vi "DBTableToTree.vi"(7 "NetworkName":string, 8 "error in (no error)":errorcluster, 9 "DBNode":T1(array[cluster]), 10 "DBSignals":T3(array[cluster]) {"SignalList"."Message_Type" items=["CAN", "CANFD", "J1939"]; "SignalList"."Mux_Type" items=["Normal", "multiplexor", "multiplexed"]; "SignalList"."Is_Motorola" items=["Intel", "Motorola"]; "SignalList"."Value_Type" items=["unsigned int", "signed int", "float", "double"]; "SignalList"."ID" format="%.0x"}, 11 "reference":refnum<vi>) -> (0 "error out":errorcluster)   [LabVIEW 2014]
uses:
  Typedef/DBSignal.ctl
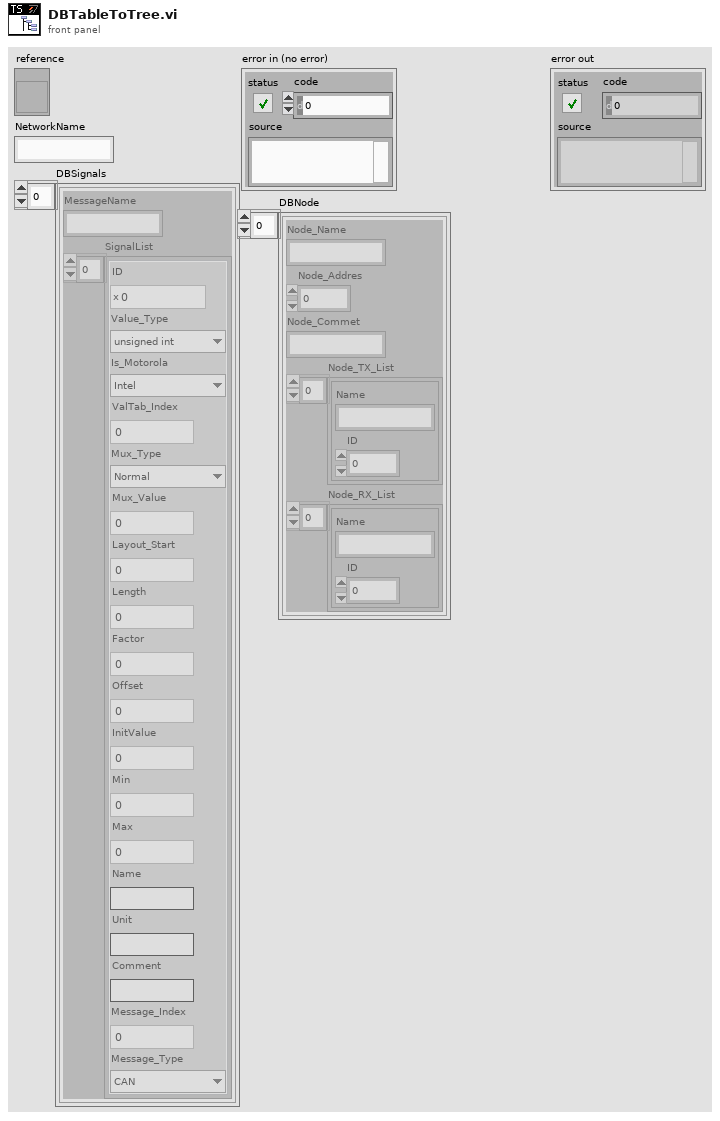
[diagram p1: front panel]
types:
  T1 = cluster{"Node_Name":string, "Node_Addres":i32, "Node_Commet":string, "Node_TX_List":cluster{"Name":string, "ID":i32}[], "Node_RX_List":cluster{"Name":string, "ID":i32}[]}[]
  T2 = typedef "DBSignal.ctl" = cluster{"ID":i32, "Value_Type":i32, "Is_Motorola":i32, "ValTab_Index":i32, "Mux_Type":i32, "Mux_Value":dbl, "Layout_Start":i32, "Length":i32, "Factor":dbl, "Offset":dbl, "InitValue":dbl, "Min":dbl, "Max":dbl, "Name":string, "Unit":string, "Comment":string, "Message_Index":i32, "Message_Type":i32}
  T3 = cluster{"MessageName":string, "SignalList":T2[]}[]
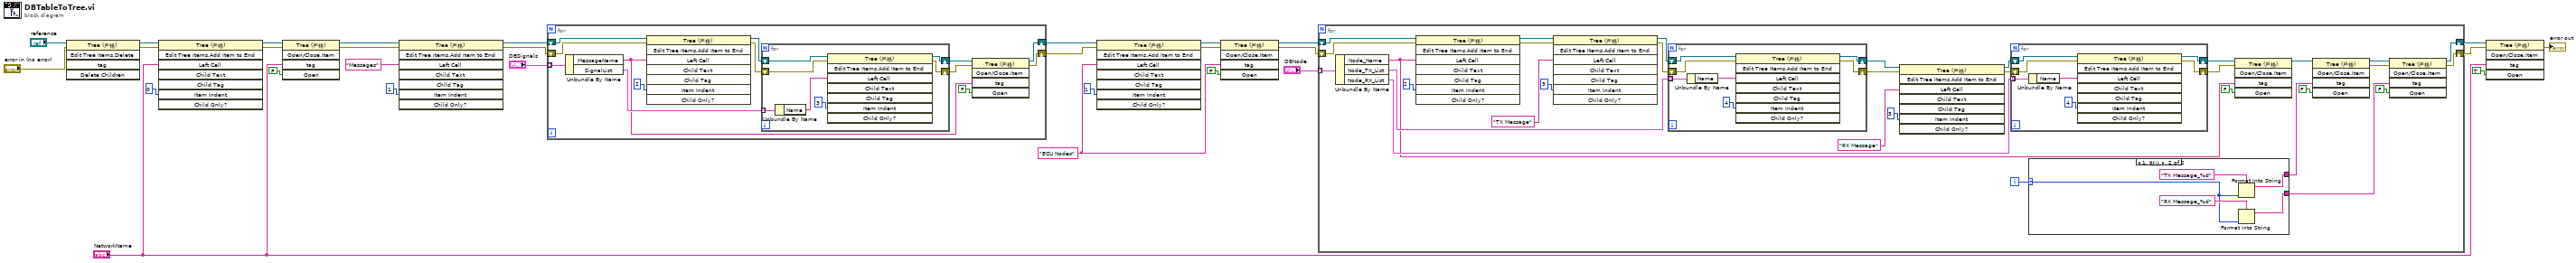
[diagram p0: block diagram]
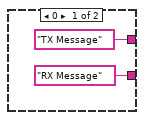
[diagram p2: hidden frame]
diagram:
  w4 = "ECU Nodes" ("Left Cell String")
  n1 = invoke class="Tree (严格)" method="Edit Tree Items.Delete"(reference="reference", error in="error in (no error)") -> (reference out=w30:refnum<vi>, error out=w18:errorcluster)  [unwired: 3 in, 3 out]
  n2 = invoke class="Tree (严格)" method="Edit Tree Items.Add Item to End"(reference=w30, error in=w18, "Left Cell"="NetworkName", "Item Indent"=0 ("New Item Indentation")) -> (reference out=w28:refnum<vi>, error out=w17:errorcluster)  [unwired: 4 in, 6 out]
  n3 = invoke class="Tree (严格)" method="Open/Close.Item"(reference=w28, error in=w17, "tag"="NetworkName", "Open"=FALSE ("Open?")) -> (reference out=w21:refnum<vi>, error out=w16:errorcluster)  [unwired: 1 in, 3 out]
  n4 = invoke class="Tree (严格)" method="Edit Tree Items.Add Item to End"(reference=w21, error in=w16, "Left Cell"="Messages" ("Left Cell String"), "Item Indent"=1 ("New Item Indentation")) -> (reference out=w15:refnum<vi>, error out=w14:errorcluster)  [unwired: 4 in, 6 out]
  n5 = for {
    tunnel: "DBSignals" -> [w42] mode=indexing
    shift-right: [w36] -> w13
    shift-left: w15 -> [w43]
    shift-right: [w31] -> w12
    shift-left: w14 -> [w34]
    n6 = Unbundle By Name(w42) -> ("MessageName"=w35:string, "SignalList"=w39:T2[])
    n7 = invoke class="Tree (严格)" method="Edit Tree Items.Add Item to End"(reference=w43, error in=w34, "Left Cell"=w35, "Item Indent"=2 ("New Item Indentation")) -> (reference out=w40:refnum<vi>, error out=w33:errorcluster)  [unwired: 4 in, 6 out]
    n8 = for {
      tunnel: w39 -> [w49] mode=indexing
      shift-right: [w46] -> w37
      shift-left: w40 -> [w50]
      shift-right: [w44] -> w32
      shift-left: w33 -> [w45]
      n9 = Unbundle By Name(w49) -> ("Name"=w48:string)
      n10 = invoke class="Tree (严格)" method="Edit Tree Items.Add Item to End"(reference=w50, error in=w45, "Left Cell"=w48, "Item Indent"=3 ("New Item Indentation")) -> (reference out=w46:refnum<vi>, error out=w44:errorcluster)  [unwired: 4 in, 6 out]
    }
    n11 = invoke class="Tree (严格)" method="Open/Close.Item"(reference=w37, error in=w32, "tag"=w35, "Open"=FALSE ("Open?")) -> (reference out=w36:refnum<vi>, error out=w31:errorcluster)  [unwired: 1 in, 3 out]
  }
  n12 = invoke class="Tree (严格)" method="Edit Tree Items.Add Item to End"(reference=w13, error in=w12, "Left Cell"=w4, "Item Indent"=1 ("New Item Indentation")) -> (reference out=w6:refnum<vi>, error out=w2:errorcluster)  [unwired: 4 in, 6 out]
  n13 = invoke class="Tree (严格)" method="Open/Close.Item"(reference=w6, error in=w2, "tag"=w4, "Open"=FALSE ("Open?")) -> (reference out=w5:refnum<vi>, error out=w1:errorcluster)  [unwired: 1 in, 3 out]
  n14 = for {
    tunnel: "DBNode" -> [w82] mode=indexing
    shift-right: [w55] -> w9
    shift-left: w5 -> [w81]
    shift-right: [w54] -> w8
    shift-left: w1 -> [w71]
    i -> [w53]
    n15 = Unbundle By Name(w82) -> ("Node_Name"=w64:string, "Node_TX_List"=w76:cluster{"Name":string, "ID":i32}[], "Node_RX_List"=w73:cluster{"Name":string, "ID":i32}[])
    n16 = invoke class="Tree (严格)" method="Edit Tree Items.Add Item to End"(reference=w81, error in=w71, "Left Cell"=w64, "Item Indent"=2 ("New Item Indentation")) -> (reference out=w79:refnum<vi>, error out=w70:errorcluster)  [unwired: 4 in, 6 out]
    n17 = invoke class="Tree (严格)" method="Edit Tree Items.Add Item to End"(reference=w79, error in=w70, "Left Cell"="TX Message" ("Left Cell String"), "Item Indent"=3 ("New Item Indentation")) -> (reference out=w77:refnum<vi>, error out=w69:errorcluster)  [unwired: 4 in, 6 out]
    n18 = for {
      tunnel: w76 -> [w95] mode=indexing
      shift-right: [w93] -> w72
      shift-left: w77 -> [w96]
      shift-right: [w90] -> w68
      shift-left: w69 -> [w91]
      n19 = Unbundle By Name(w95) -> ("Name"=w94:string)
      n20 = invoke class="Tree (严格)" method="Edit Tree Items.Add Item to End"(reference=w96, error in=w91, "Left Cell"=w94, "Item Indent"=4 ("New Item Indentation")) -> (reference out=w93:refnum<vi>, error out=w90:errorcluster)  [unwired: 4 in, 6 out]
    }
    n21 = invoke class="Tree (严格)" method="Edit Tree Items.Add Item to End"(reference=w72, error in=w68, "Left Cell"="RX Message" ("Left Cell String"), "Item Indent"=3 ("New Item Indentation")) -> (reference out=w75:refnum<vi>, error out=w67:errorcluster)  [unwired: 4 in, 6 out]
    n22 = for {
      tunnel: w73 -> [w102] mode=indexing
      shift-right: [w100] -> w66
      shift-left: w75 -> [w103]
      shift-right: [w97] -> w65
      shift-left: w67 -> [w98]
      n23 = Unbundle By Name(w102) -> ("Name"=w101:string)
      n24 = invoke class="Tree (严格)" method="Edit Tree Items.Add Item to End"(reference=w103, error in=w98, "Left Cell"=w101, "Item Indent"=4 ("New Item Indentation")) -> (reference out=w100:refnum<vi>, error out=w97:errorcluster)  [unwired: 4 in, 6 out]
    }
    n25 = case shown="1, 默认" w53 {
      selector: w53 -> [_ w87]
      tunnel: ["TX Message" ("Left Cell String") w86] -> w52
      tunnel: ["RX Message" ("Left Cell String") w85] -> w51
      frame 0 {
      }
      frame 1, Default {
        n26 = Format Into String(format string="TX Message_%d", w87) -> (resulting string=w86:string)  [unwired: 2 in, 1 out]
        n27 = Format Into String(format string="RX Message_%d", w87) -> (resulting string=w85:string)  [unwired: 2 in, 1 out]
      }
    }
    n28 = invoke class="Tree (严格)" method="Open/Close.Item"(reference=w66, error in=w65, "tag"=w64, "Open"=FALSE ("Open?")) -> (reference out=w62:refnum<vi>)  [unwired: 1 in, 4 out]
    n29 = invoke class="Tree (严格)" method="Open/Close.Item"(reference=w62, "tag"=w52, "Open"=FALSE ("Open?")) -> (reference out=w60:refnum<vi>, error out=w59:errorcluster)  [unwired: 2 in, 3 out]
    n30 = invoke class="Tree (严格)" method="Open/Close.Item"(reference=w60, error in=w59, "tag"=w51, "Open"=FALSE ("Open?")) -> (reference out=w55:refnum<vi>, error out=w54:errorcluster)  [unwired: 1 in, 3 out]
  }
  n31 = invoke class="Tree (严格)" method="Open/Close.Item"(reference=w9, error in=w8, "tag"="NetworkName", "Open"=TRUE ("Open?")) -> (error out=→"error out":errorcluster)  [unwired: 1 in, 4 out]
